vi "createCommandInputStr.vi"(8 "error in (no error)":errorcluster, 9 "dataType":T1, 10 "data":variant, 11 "CoolerSerialCommand in":refnum<class "CoolerSerialCommand.lvclass">) -> (0 "error out":errorcluster, 2 "cmdDataStr":string, 3 "CoolerSerialCommand out":refnum<class "CoolerSerialCommand.lvclass">)   [LabVIEW 2016, in "CoolerSerialCommand.lvclass"]
uses:
  CoolerSerialCommand.lvclass
  typedefs/dataType.ctl
  typedefs/ControlSensor.ctl
  typedefs/ExternalSensorStatus.ctl
  typedefs/ChillerStatus.ctl
panel:
  out "length":i32
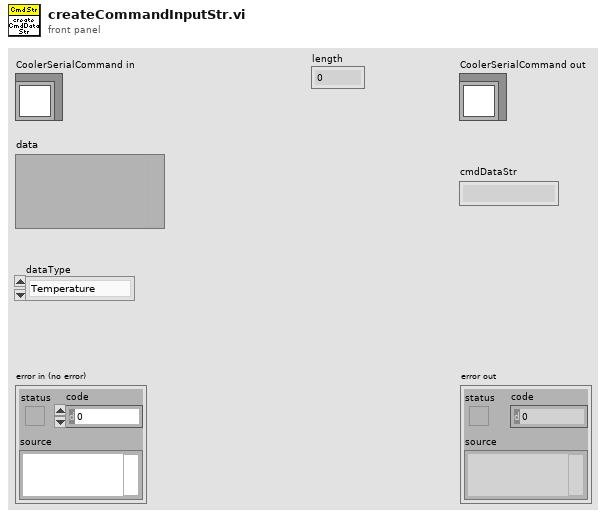
[diagram p1: front panel]
types:
  T1 = typedef "dataType.ctl" = enum16{"Temperature", "Flow", "ControlSensor", "ExternalSensorStatus", "ChillerStatus"}
  T2 = typedef "ControlSensor.ctl" = enum16{"SupplyTemperature", "ReturnTemperature", "ExtRTD", "ExternalTermistor"}
  T3 = typedef "ExternalSensorStatus.ctl" = enum16{"Disabled", "Enabled"}
  T4 = typedef "ChillerStatus.ctl" = enum16{"StandBy", "Run"}
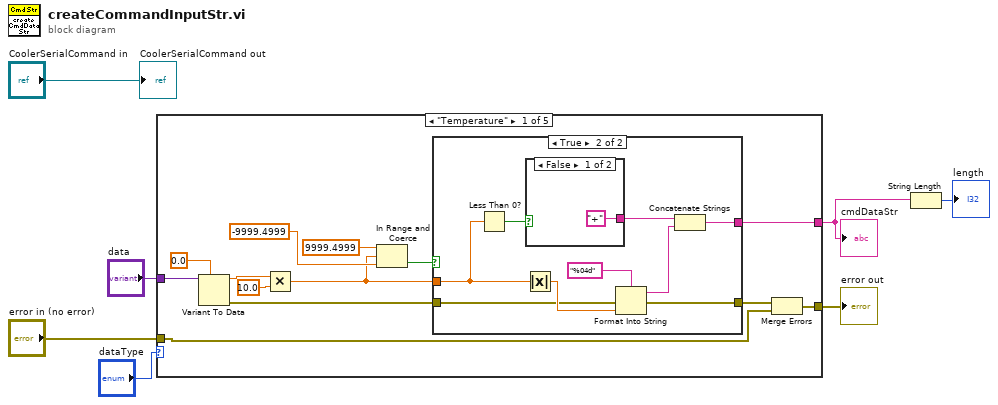
[diagram p0: block diagram]
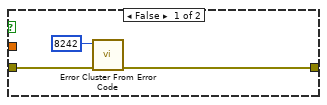
[diagram p2: hidden frame]
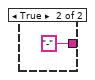
[diagram p3: hidden frame]
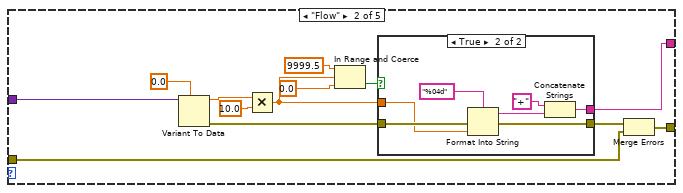
[diagram p4: hidden frame]
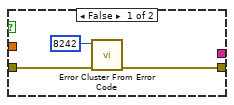
[diagram p5: hidden frame]
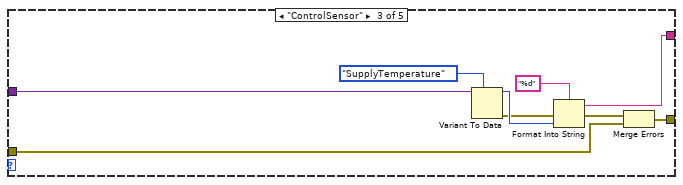
[diagram p6: hidden frame]
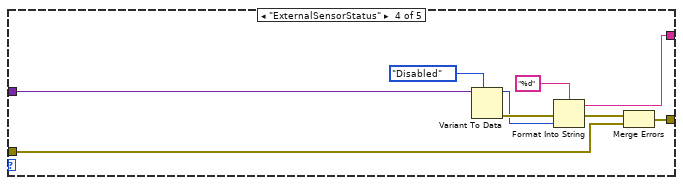
[diagram p7: hidden frame]
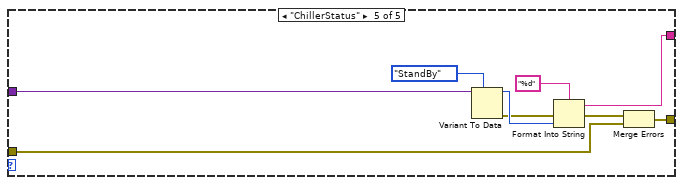
[diagram p8: hidden frame]
diagram:
  n1 = case shown="\"Temperature\"" "dataType" {
    tunnel: "data" -> [w20 w47 w66 w75 w84]
    tunnel: "error in (no error)" -> [w11 w38 w61 w69 w76]
    tunnel: [w17 w45 w62 w70 w79] -> w1
    tunnel: [w8 w35 w59 w67 w78] -> w2
    frame "Temperature" {
      n2 = Variant To Data(type=0.0, Variant=w20) -> (data=w13:dbl, error out=w10:errorcluster)  [unwired: 1 in]
      n3 = Multiply(x=w13, y=10.0) -> (x*y=w12:dbl)
      n4 = In Range and Coerce(upper limit=9999.4999, x=w12, lower limit=-9999.4999) -> (In Range?=w14:bool)  [unwired: 1 out]
      n5 = case shown="True" w14 {
        tunnel: [_ w24] -> w17
        tunnel: w12 -> [_ w25]
        tunnel: w10 -> [w22 w27]
        tunnel: [w21 w26] -> w9
        frame False {
          n6 = call <vilib>:"Error Cluster From Error Code.vi"("error in (no error)"=w22, "error code (0)"=8242) -> ("error out"=w21:errorcluster)  [unwired: 7 in]
        }
        frame True {
          n7 = Less Than 0?(x=w25) -> (x < 0?=w30:bool)
          n8 = Absolute Value(x=w25) -> (abs(x)=w28:dbl)
          n9 = case shown="False" w30 {
            tunnel: ["+" ("string") "-" ("string")] -> w29
            frame False {
            }
            frame True {
            }
          }
          n10 = Format Into String(format string="%04d", error in=w27, w28) -> (resulting string=w31:string, error out=w26:errorcluster)  [unwired: 1 in]
          n11 = Concatenate Strings(w29, w31) -> (w24:string)
        }
      }
      n12 = Merge Errors(w9, w11) -> (w8:errorcluster)
    }
    frame "Flow" {
      n13 = Variant To Data(type=0.0, Variant=w47) -> (data=w43:dbl, error out=w37:errorcluster)  [unwired: 1 in]
      n14 = Multiply(x=w43, y=10.0) -> (x*y=w42:dbl)
      n15 = In Range and Coerce(upper limit=9999.5, x=w42, lower limit=0.0) -> (In Range?=w39:bool)  [unwired: 1 out]
      n16 = case shown="True" w39 {
        tunnel: w37 -> [w50 w56]
        tunnel: [w49 w55] -> w36
        tunnel: [_ w53] -> w45
        tunnel: w42 -> [_ w51]
        frame False {
          n17 = call <vilib>:"Error Cluster From Error Code.vi"("error in (no error)"=w50, "error code (0)"=8242) -> ("error out"=w49:errorcluster)  [unwired: 7 in]
        }
        frame True {
          n18 = Format Into String(format string="%04d", error in=w56, w51) -> (resulting string=w54:string, error out=w55:errorcluster)  [unwired: 1 in]
          n19 = Concatenate Strings("+" ("string"), w54) -> (w53:string)
        }
      }
      n20 = Merge Errors(w36, w38) -> (w35:errorcluster)
    }
    frame "ControlSensor" {
      n21 = Variant To Data(type=ControlSensor."SupplyTemperature" ("ControlSensor"), Variant=w66) -> (data=w64:T2, error out=w58:errorcluster)  [unwired: 1 in]
      n22 = Format Into String(format string="%d", error in=w58, w64) -> (resulting string=w62:string, error out=w60:errorcluster)  [unwired: 1 in]
      n23 = Merge Errors(w60, w61) -> (w59:errorcluster)
    }
    frame "ExternalSensorStatus" {
      n24 = Variant To Data(type=ExternalSensorStatus."Disabled" ("ExternalSensorStatus"), Variant=w75) -> (data=w71:T3, error out=w72:errorcluster)  [unwired: 1 in]
      n25 = Format Into String(format string="%d", error in=w72, w71) -> (resulting string=w70:string, error out=w68:errorcluster)  [unwired: 1 in]
      n26 = Merge Errors(w68, w69) -> (w67:errorcluster)
    }
    frame "ChillerStatus" {
      n27 = Variant To Data(type=ChillerStatus."StandBy" ("ChillerStatus"), Variant=w84) -> (data=w81:T4, error out=w80:errorcluster)  [unwired: 1 in]
      n28 = Format Into String(format string="%d", error in=w80, w81) -> (resulting string=w79:string, error out=w77:errorcluster)  [unwired: 1 in]
      n29 = Merge Errors(w77, w76) -> (w78:errorcluster)
    }
  }
  "error out" <- w2
  "cmdDataStr" <- w1
  n30 = String Length(string=w1) -> (length=→"length":i32)
  "CoolerSerialCommand out" <- "CoolerSerialCommand in"
